vi "Make_Source_Item.vi"(8 "error in (no error)":errorcluster, 10 "IB_Destination.lvclass":refnum<class "IB_Destination.lvclass">, 11 "IB_Tree_Item_Proj_CGen in":refnum<class "IB_Tree_Item_Proj_CGen.lvclass">) -> (0 "error out":errorcluster, 3 "IB_Source.lvclass":refnum<class "IB_Source.lvclass">)   [LabVIEW 2020, in "IB_Tree_Item_Proj_CGen.lvclass"]
uses:
  <vilib>/AppBuilder/IB_Classes/Tree_Item_Proj_CGen/IB_Tree_Item_Proj_CGen.lvclass
  <vilib>/AppBuilder/IB_Classes/Tree_Item_Proj_CGen/IB_Tree_Item_Proj_CGen.lvclass/IB_Tree_Item_Proj_CGen.ctl
  <vilib>/AppBuilder/IB_Classes/Source/Container/Build/CGen/IB_CGen.lvclass
  e:/builds/penguin/labview/branches/2020/dev/dist/vi.lib/AppBuilder/IB_Classes/Tree_Item_Proj_Build/IB_Tree_Item_Proj_Build.lvclass
  e:/builds/penguin/labview/branches/2020/dev/dist/vi.lib/AppBuilder/IB_Classes/Tree_Item_Proj_Container/IB_Tree_Item_Proj_Container.lvclass
  e:/builds/penguin/labview/branches/2020/dev/dist/vi.lib/AppBuilder/IB_Classes/Tree_Item_Proj/IB_Tree_Item_Proj.lvclass
  e:/builds/penguin/labview/branches/2020/dev/dist/vi.lib/AppBuilder/IB_Classes/Tree_Item/IB_Tree_Item.lvclass
  e:/builds/penguin/labview/branches/2020/dev/dist/vi.lib/AppBuilder/IB_Classes/Tree_Item_Proj_CGen/IB_Tree_Item_Proj_CGen.lvclass
  e:/builds/penguin/labview/branches/2020/dev/dist/vi.lib/AppBuilder/IB_Classes/Source/Container/Build/IB_Source_Build.lvclass
  e:/builds/penguin/labview/branches/2020/dev/dist/vi.lib/AppBuilder/IB_Classes/Source/Container/IB_Source_Container.lvclass
  e:/builds/penguin/labview/branches/2020/dev/dist/vi.lib/AppBuilder/IB_Classes/Source/IB_Source.lvclass
  e:/builds/penguin/labview/branches/2020/dev/dist/vi.lib/AppBuilder/IB_Classes/Source/Container/Build/CGen/IB_CGen.lvclass
  <vilib>/AppBuilder/IB_Classes/Source/IB_Source.lvclass
  <vilib>/AppBuilder/IB_Classes/Destination/IB_Destination.lvclass
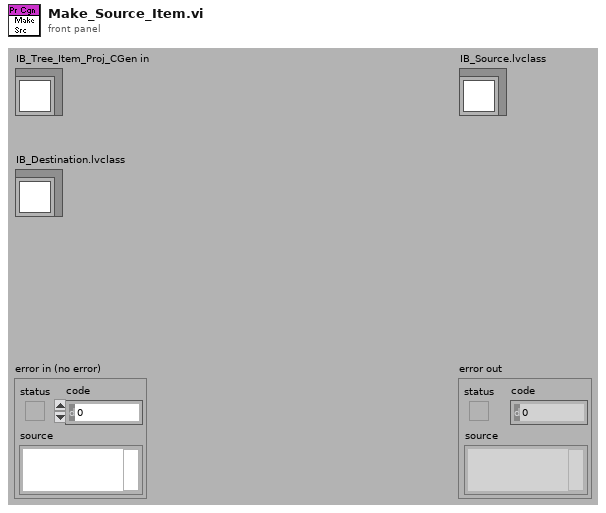
[diagram p1: front panel]
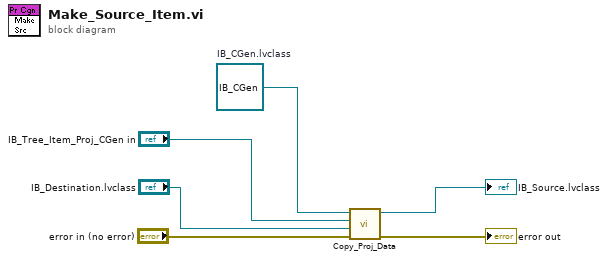
[diagram p0: block diagram]
diagram:
  w1 = refnum<class "IB_CGen.lvclass"> refnum  # IB_CGen.lvclass
  n1 = call-dynamic "Copy_Proj_Data.vi"("error in (no error)"="error in (no error)", "IB_Destination.lvclass"="IB_Destination.lvclass", "IB_Tree_Item_Proj in"="IB_Tree_Item_Proj_CGen in", "IB_Source_Build in"=w1) -> ("error out"=→"error out":errorcluster, "IB_Source_Build out"=→"IB_Source.lvclass":refnum<class "IB_CGen.lvclass">)  [unwired: 6 out]
